vi "Maps-Marker.vi"(0 "Google Maps Resource Out in":T2, 7 "Marker":T1, 11 "error in (no error)":errorcluster) -> (4 "Google Maps Resource Out out":T2, 15 "error out":errorcluster)   [LabVIEW 2020]
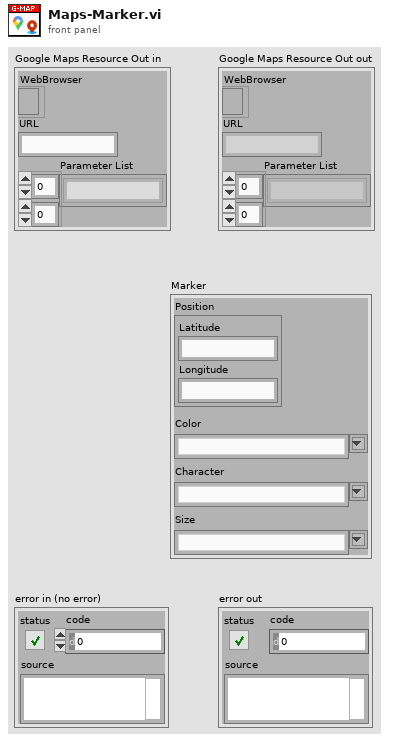
[diagram p1: front panel]
types:
  T1 = cluster{"Position":cluster{"Latitude":string, "Longitude":string}, "Color":string, "Character":string, "Size":string}
  T2 = cluster{"WebBrowser":refnum<k7>, "URL":string, "Parameter List":string[][]}
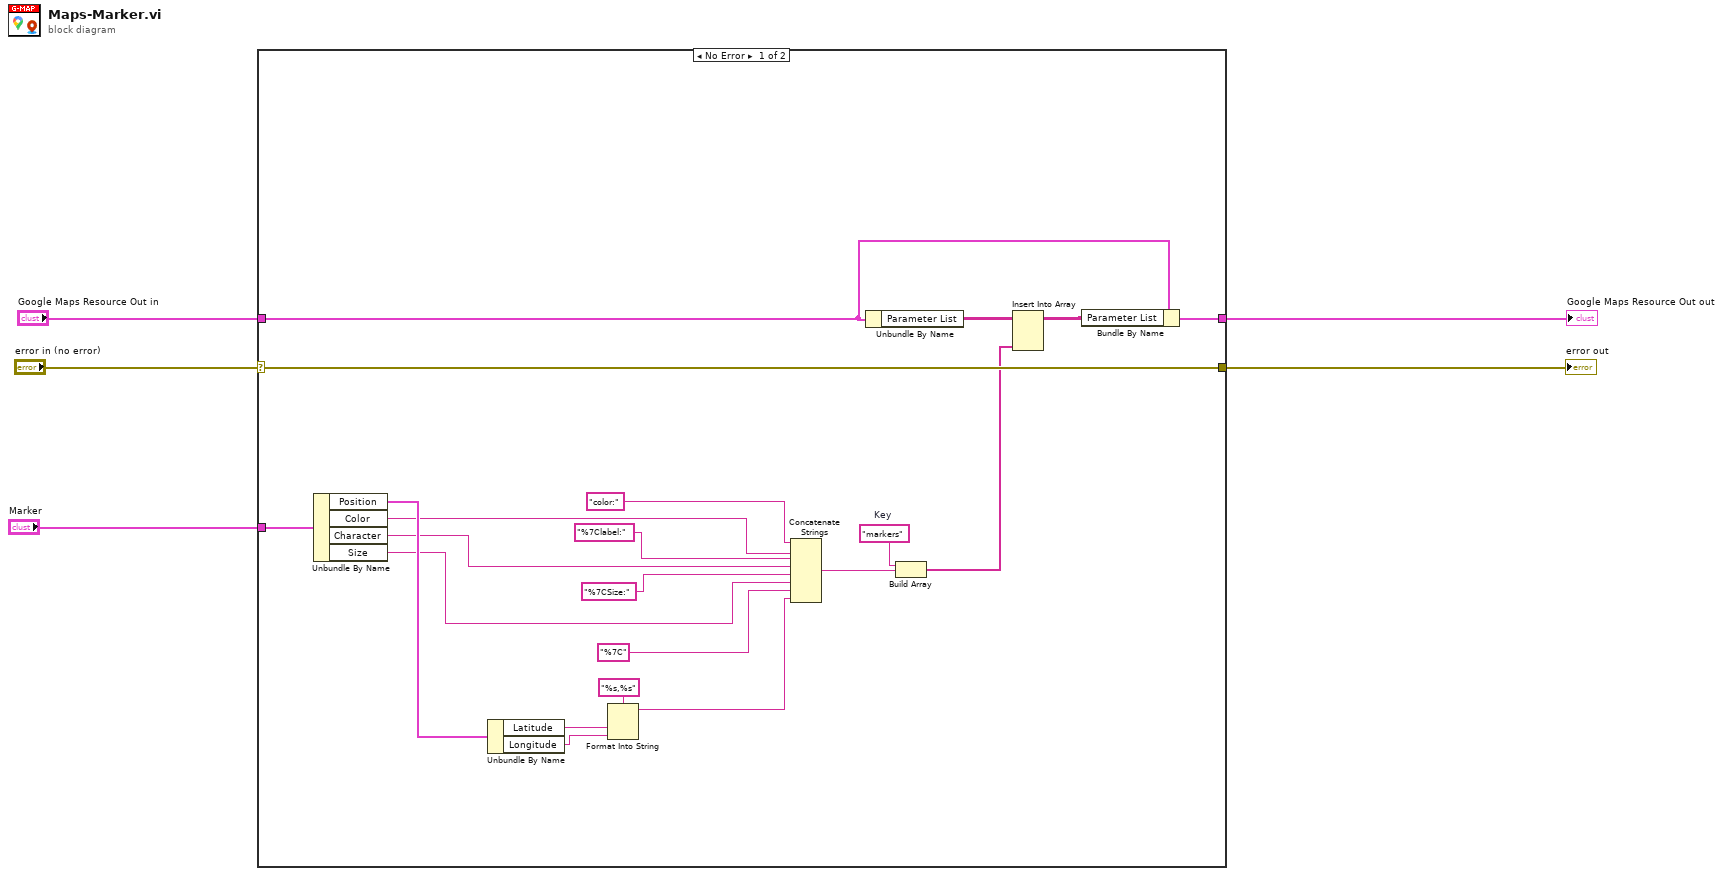
[diagram p0: block diagram]
diagram:
  n1 = case shown="No Error" "error in (no error)" {
    selector: "error in (no error)" -> [w26 w27]
    tunnel: "Google Maps Resource Out in" -> [w9 w28]
    tunnel: [w8 w28] -> w3
    tunnel: [w26 w27] -> w5
    tunnel: "Marker" -> [w13 _]
    frame No Error {
      w7 = "markers"  # Key
      n2 = Unbundle By Name(w13) -> ("Position"=w22:cluster{"Latitude":string, "Longitude":string}, "Color"=w21:string, "Character"=w20:string, "Size"=w19:string)
      n3 = Unbundle By Name(w22) -> ("Latitude"=w25:string, "Longitude"=w24:string)
      n4 = Format Into String(format string="%s,%s", w25, w24) -> (resulting string=w23:string)  [unwired: 2 in, 1 out]
      n5 = Concatenate Strings("color:", w21, "%7Clabel:" ("string"), w20, "%7CSize:" ("string"), w19, "%7C" ("string"), w23) -> (w6:string)
      n6 = Unbundle By Name(w9) -> ("Parameter List"=w10:string[][])
      n7 = Build Array(w7, w6) -> (w11:string[])
      n8 = Insert Into Array(array=w10, new element=w11) -> (w12:string[][])  [unwired: 2 in]
      n9 = Bundle By Name(cluster=w9, "Parameter List"=w12) -> (w8:T2)
    }
    frame Error {
    }
  }
  "error out" <- w5
  "Google Maps Resource Out out" <- w3
